vi "数组降维.vi"() -> ()   [LabVIEW 2018]
panel:
  in  "添加的数组":bool[][](array[boolean])
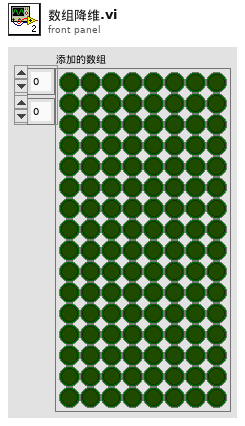
[diagram p1: front panel]
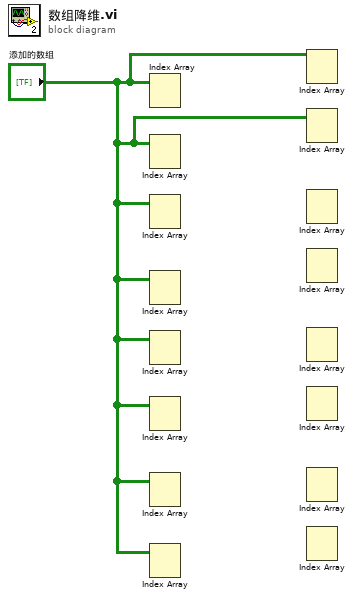
[diagram p0: block diagram]
diagram:
  n1 = Index Array(array="添加的数组") -> ()  [unwired: 2 in, 1 out]
  n2 = Index Array(array="添加的数组") -> ()  [unwired: 2 in, 1 out]
  n3 = Index Array(array="添加的数组") -> ()  [unwired: 2 in, 1 out]
  n4 = Index Array(array="添加的数组") -> ()  [unwired: 2 in, 1 out]
  n5 = Index Array(array="添加的数组") -> ()  [unwired: 2 in, 1 out]
  n6 = Index Array(array="添加的数组") -> ()  [unwired: 2 in, 1 out]
  n7 = Index Array(array="添加的数组") -> ()  [unwired: 2 in, 1 out]
  n8 = Index Array(array="添加的数组") -> ()  [unwired: 2 in, 1 out]
  n9 = Index Array(array="添加的数组") -> ()  [unwired: 2 in, 1 out]
  n10 = Index Array(array="添加的数组") -> ()  [unwired: 2 in, 1 out]
  n11 = Index Array() -> ()  [unwired: 3 in, 1 out]
  n12 = Index Array() -> ()  [unwired: 3 in, 1 out]
  n13 = Index Array() -> ()  [unwired: 3 in, 1 out]
  n14 = Index Array() -> ()  [unwired: 3 in, 1 out]
  n15 = Index Array() -> ()  [unwired: 3 in, 1 out]
  n16 = Index Array() -> ()  [unwired: 3 in, 1 out]
